vi "_PC_Daemon_MSConf_AccessParam.vi"(7 "Function":enum16{"Write", "Read"}(ring), 8 "error in (no error)":errorcluster, 11 "Execution.Param in":T2={"Method"=path "", "Loops"=1, "AVG"=1, "ContinuesRun"=FALSE}) -> (0 "error out":errorcluster, 3 "exe param memory":T1)   [LabVIEW 2018]
uses:
  PublicSubVI/Ctl/RegistyFunc.ctl
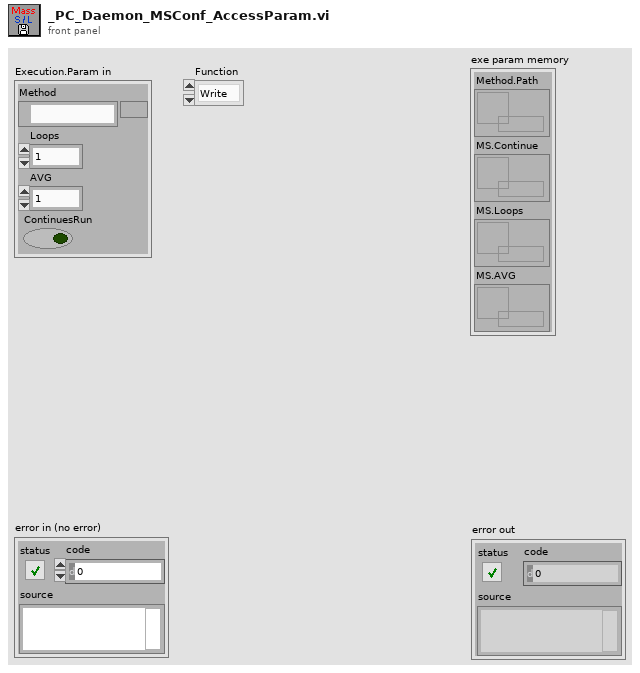
[diagram p1: front panel]
types:
  T1 = cluster{"Method.Path":refnum<data-value>, "MS.Continue":refnum<data-value>, "MS.Loops":refnum<data-value>, "MS.AVG":refnum<data-value>}
  T2 = cluster{"Method":path, "Loops":i32, "AVG":u8, "ContinuesRun":bool}
  T3 = typedef "RegistyFunc.ctl" = enum16{"None", "FileAutoSave", "FileNoise", "FileSN", "ExeStatu", "WorkFolderPath", "MethodPath", "AVGItem", "LoopItem", "AutoRun", "BGColor", "LineColor", "LineWidth", "XGrid", "YGrid", "DeviceRefnum"}
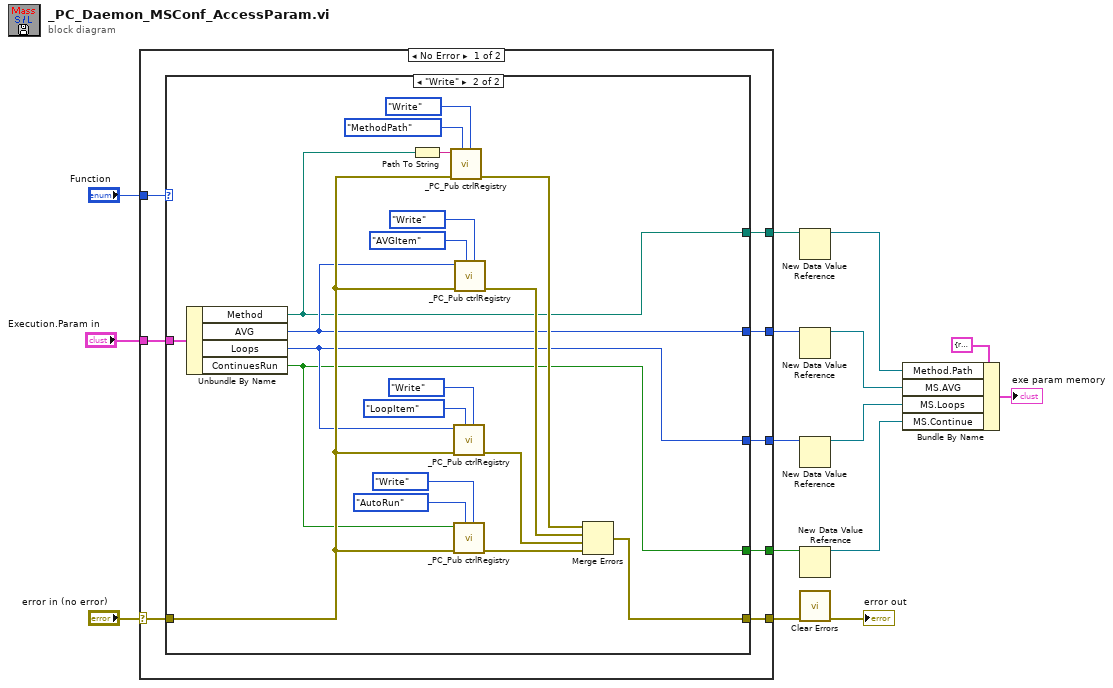
[diagram p0: block diagram]
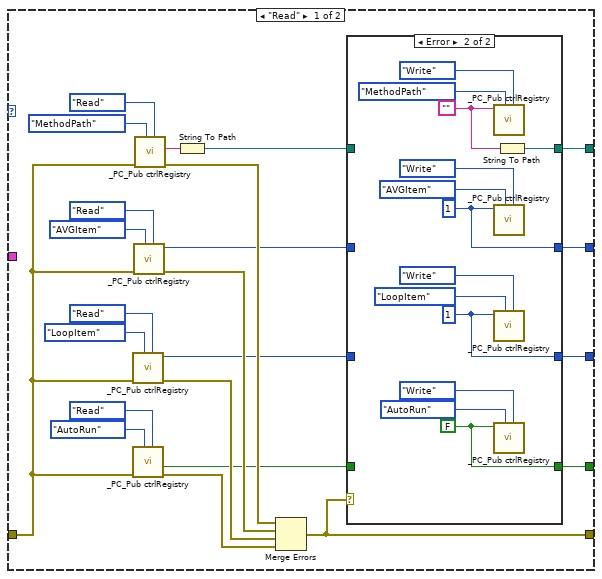
[diagram p2: hidden frame]
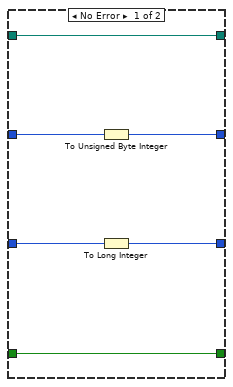
[diagram p3: hidden frame]
diagram:
  n1 = case shown="No Error" "error in (no error)" {
    selector: "error in (no error)" -> [w20 w86]
    tunnel: "Function" -> [w23 _]
    tunnel: "Execution.Param in" -> [w22 _]
    tunnel: [w21 w86] -> w13
    tunnel: [w19 _] -> w10
    tunnel: [w18 _] -> w7
    tunnel: [w17 _] -> w8
    tunnel: [w16 _] -> w9
    frame No Error {
      n2 = case shown="\"Write\"" w23 {
        tunnel: [w28 w73] -> w21
        tunnel: w22 -> [_ w71]
        tunnel: w20 -> [w34 w72]
        tunnel: [w27 w67] -> w19
        tunnel: [w26 w68] -> w18
        tunnel: [w25 w69] -> w17
        tunnel: [w24 w66] -> w16
        frame "Read" {
          n3 = call "_PC_Pub ctrlRegistry.vi"("type"=enum16{"None", "Write", "Read"}."Read", "function"=RegistyFunc."LoopItem", "error in (no error)"=w34) -> ("error out"=w45:errorcluster, "DWORD outpur"=w30:u32)  [unwired: 5 in, 2 out]
          n4 = call "_PC_Pub ctrlRegistry.vi"("type"=enum16{"None", "Write", "Read"}."Read", "function"=RegistyFunc."AutoRun", "error in (no error)"=w34) -> ("error out"=w46:errorcluster, "Boolean output"=w29:bool)  [unwired: 5 in, 2 out]
          n5 = call "_PC_Pub ctrlRegistry.vi"("type"=enum16{"None", "Write", "Read"}."Read", "function"=RegistyFunc."AVGItem", "error in (no error)"=w34) -> ("error out"=w44:errorcluster, "DWORD outpur"=w31:u32)  [unwired: 5 in, 2 out]
          n6 = call "_PC_Pub ctrlRegistry.vi"("type"=enum16{"None", "Write", "Read"}."Read", "function"=RegistyFunc."MethodPath", "error in (no error)"=w34) -> ("error out"=w43:errorcluster, "SZ output"=w33:string)  [unwired: 5 in, 2 out]
          n7 = String To Path(string=w33) -> (path=w32:path)
          n8 = Merge Errors(w43, w44, w45, w46) -> (w28:errorcluster)
          n9 = case shown="Error" w28 {
            tunnel: w32 -> [w52 _]
            tunnel: w31 -> [w51 _]
            tunnel: w30 -> [w50 _]
            tunnel: w29 -> [w49 _]
            tunnel: [w49 w57] -> w27
            tunnel: [w47 w56] -> w26
            tunnel: [w48 w55] -> w25
            tunnel: [w52 w53] -> w24
            frame No Error {
              n10 = To Unsigned Byte Integer(number=w51) -> (unsigned 8bit integer=w48:u8)
              n11 = To Long Integer(number=w50) -> (32bit integer=w47:i32)
            }
            frame Error {
              w57 = FALSE ("ContinuesRun")
              w56 = 1 ("AVG")
              w55 = u8 1 ("Loops")
              w54 = ""
              n12 = call "_PC_Pub ctrlRegistry.vi"("type"=enum16{"None", "Write", "Read"}."Write", "function"=RegistyFunc."MethodPath", "write value"=w54) -> ()  [unwired: 5 in, 4 out]
              n13 = call "_PC_Pub ctrlRegistry.vi"("type"=enum16{"None", "Write", "Read"}."Write", "function"=RegistyFunc."AVGItem", "write value"=w55) -> ()  [unwired: 5 in, 4 out]
              n14 = call "_PC_Pub ctrlRegistry.vi"("type"=enum16{"None", "Write", "Read"}."Write", "function"=RegistyFunc."LoopItem", "write value"=w56) -> ()  [unwired: 5 in, 4 out]
              n15 = call "_PC_Pub ctrlRegistry.vi"("type"=enum16{"None", "Write", "Read"}."Write", "function"=RegistyFunc."AutoRun", "write value"=w57) -> ()  [unwired: 5 in, 4 out]
              n16 = String To Path(string=w54) -> (path=w53:path)
            }
          }
        }
        frame "Write" {
          n17 = Unbundle By Name(w71) -> ("Method"=w66:path, "AVG"=w69:u8, "Loops"=w68:i32, "ContinuesRun"=w67:bool)
          n18 = Path To String(path=w66) -> (string=w70:string)
          n19 = call "_PC_Pub ctrlRegistry.vi"("type"=enum16{"None", "Write", "Read"}."Write", "function"=RegistyFunc."MethodPath", "error in (no error)"=w72, "write value"=w70) -> ("error out"=w82:errorcluster)  [unwired: 4 in, 3 out]
          n20 = call "_PC_Pub ctrlRegistry.vi"("type"=enum16{"None", "Write", "Read"}."Write", "function"=RegistyFunc."LoopItem", "error in (no error)"=w72, "write value"=w68) -> ("error out"=w84:errorcluster)  [unwired: 4 in, 3 out]
          n21 = call "_PC_Pub ctrlRegistry.vi"("type"=enum16{"None", "Write", "Read"}."Write", "function"=RegistyFunc."AutoRun", "error in (no error)"=w72, "write value"=w67) -> ("error out"=w85:errorcluster)  [unwired: 4 in, 3 out]
          n22 = call "_PC_Pub ctrlRegistry.vi"("type"=enum16{"None", "Write", "Read"}."Write", "function"=RegistyFunc."AVGItem", "error in (no error)"=w72, "write value"=w69) -> ("error out"=w83:errorcluster)  [unwired: 4 in, 3 out]
          n23 = Merge Errors(w82, w83, w84, w85) -> (w73:errorcluster)
        }
      }
    }
    frame Error {
    }
  }
  n24 = New Data Value Reference(data value=w9) -> (data value reference=w5:refnum<data-value>)  [unwired: 1 in, 1 out]
  n25 = New Data Value Reference(data value=w8) -> (data value reference=w4:refnum<data-value>)  [unwired: 1 in, 1 out]
  n26 = New Data Value Reference(data value=w7) -> (data value reference=w2:refnum<data-value>)  [unwired: 1 in, 1 out]
  n27 = New Data Value Reference(data value=w10) -> (data value reference=w3:refnum<data-value>)  [unwired: 1 in, 1 out]
  n28 = call <vilib>:"Clear Errors.vi"("error in (no error)"=w13) -> ("error out"=→"error out":errorcluster)  [unwired: 5 in, 1 out]
  n29 = Bundle By Name(cluster=T1 {"Method.Path"=refnum, "MS.Continue"=refnum, "MS.Loops"=refnum, "MS.AVG"=refnum}, "Method.Path"=w5, "MS.AVG"=w4, "MS.Loops"=w2, "MS.Continue"=w3) -> (→"exe param memory":T1)
